vi "mxwScript_Cmnd2Str_runVIOnObject.vi"(8 "error in (no error)":errorcluster, 11 "data":variant) -> (0 "error out":errorcluster, 3 "outputString":string)   [LabVIEW 2017]
uses:
  codeGenAPISupport.llb/cgAPI_mxwScript_RunVIOnObjectInfo.ctl
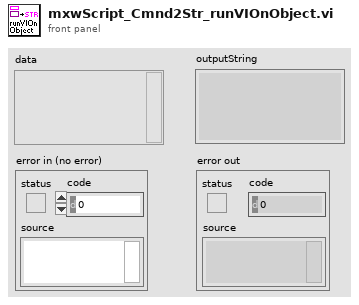
[diagram p1: front panel]
types:
  T1 = typedef "cgAPI_mxwScript_RunVIOnObjectInfo.ctl" = cluster{"name":string, "context":string, "viPath":path, "synch":bool, "parameters":cluster{"label":string, "value":variant}[], "modifyStack?":bool}
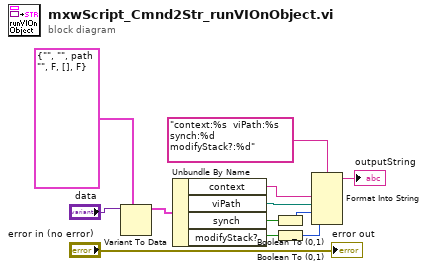
[diagram p0: block diagram]
diagram:
  n1 = Variant To Data(type=T1 {"name"="", "context"="", "viPath"=path "", "synch"=FALSE, "parameters"=[], "modifyStack?"=FALSE} ("RunVIOnObject info"), Variant="data") -> (data=w10:T1)  [unwired: 1 in, 1 out]
  n2 = Unbundle By Name(w10) -> ("context"=w7:string, "viPath"=w8:path, "synch"=w4:bool, "modifyStack?"=w2:bool)
  n3 = Boolean To (0,1)(Boolean=w4) -> (0, 1=w1:i16)
  n4 = Boolean To (0,1)(Boolean=w2) -> (0, 1=w3:i16)
  n5 = Format Into String(format string="context:%s  viPath:%s  synch:%d  modifyStack?:%d", w7, w8, w1, w3) -> (resulting string=→"outputString":string)  [unwired: 2 in, 1 out]
  "error out" <- "error in (no error)"
